vi "采配水流程与超标留样交互.vi"(11 "参数":T1) -> ()   [LabVIEW 2016, in "PLC.lvlib"]
uses:
  PLC.lvlib
panel:
  out "输出数组":cluster{"参数名":string, "浓度":dbl}[](array[cluster])
  out "数值":i32
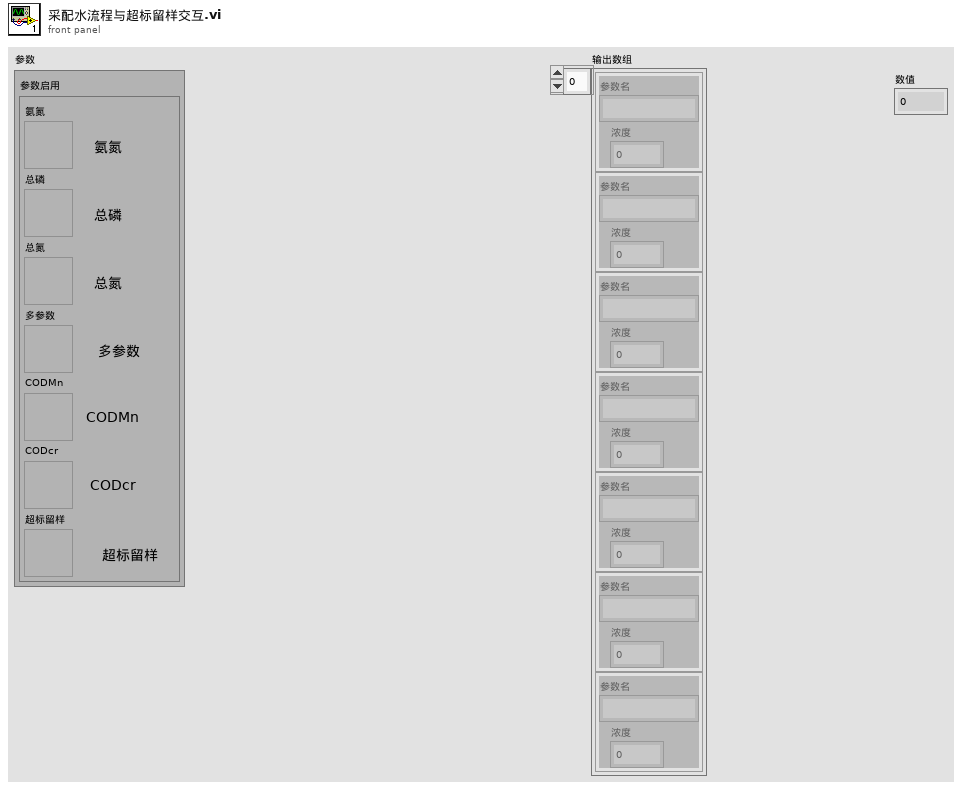
[diagram p1: front panel]
types:
  T1 = cluster{"参数启用":cluster{"氨氮":bool, "总磷":bool, "总氮":bool, "多参数":bool, "CODMn":bool, "CODcr":bool, "超标留样":bool}}
  T2 = cluster{"因子编码":u32, "单位":u16, "标样参考值":sgl, "水样数据时间":timestamp, "水样实测值":sgl, "水样数据标识":string, "标样数据时间":timestamp, "标样实测值":sgl, "标样数据标识":string, "空白数据时间":timestamp, "空白实测值":sgl, "空白数据标识":string, "零点核查数据时间":timestamp, "零点核查实测值":sgl, "零点核查数据标识":string, "跨度核查数据时间":timestamp, "跨度核查实测值":sgl, "跨度核查数据标识":string, "加标回收数据时间":timestamp, "加标回收实测值":sgl, "加标回收数据标识":string, "平行样数据时间":timestamp, "平行样实测值":sgl, "平行样数据标识":string, "F0":sgl, "F1":sgl, "F2":sgl, "F3":sgl, "F4":sgl, "F5":sgl, "F6":sgl, "F7":sgl, "温度":sgl, "湿度":sgl, "X值":sgl, "fidrange":u16}
  T3 = cluster{"温度测量值":sgl, "测量值":sgl, "温度偏移修正值":sgl, "信号值":sgl, "数据标识":string}
  T4 = cluster{"温度测量值":sgl, "DO%":sgl, "DOmg/L":sgl, "温度偏移修正值":sgl, "数据标识mg/L":string, "数据标识%":string}
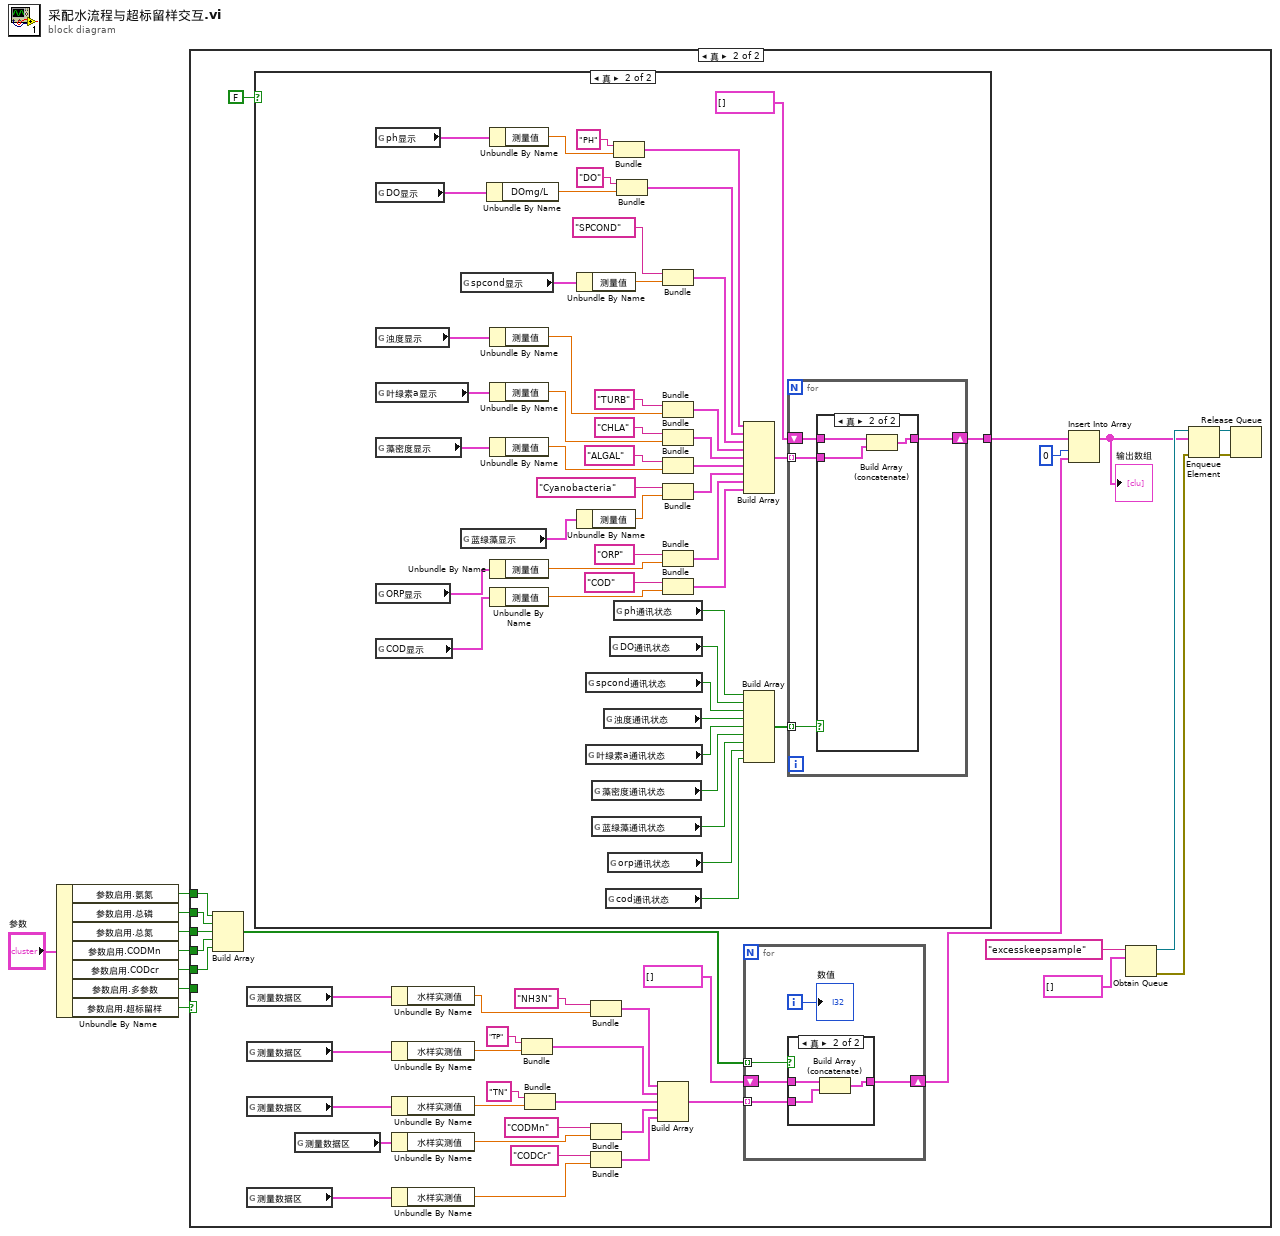
[diagram p0: block diagram]
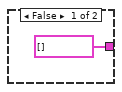
[diagram p4: hidden frame]
diagram:
  n1 = Unbundle By Name("参数") -> ("参数启用.氨氮"=w2:bool, "参数启用.总磷"=w3:bool, "参数启用.总氮"=w4:bool, "参数启用.CODMn"=w5:bool, "参数启用.CODcr"=w6:bool, "参数启用.多参数"=w7:bool, "参数启用.超标留样"=w1:bool)
  n2 = case shown="真" w1 {
    tunnel: w7 -> [_ _]
    tunnel: w6 -> [_ w33]
    tunnel: w5 -> [_ w32]
    tunnel: w4 -> [_ w31]
    tunnel: w3 -> [_ w30]
    tunnel: w2 -> [_ w29]
    frame False {
    }
    frame True {
      n3 = Build Array(w29, w30, w31, w32, w33) -> (w28:bool[])
      n4 = global read "VAR总磷总氮全局变量.vi" "测量数据区"() -> (w40:T2)
      n5 = global read "VAR总磷总氮全局变量.vi" "测量数据区"() -> (w35:T2)
      n6 = global read "VAR总磷总氮全局变量.vi" "测量数据区"() -> (w34:T2)
      n7 = global read "VAR总磷总氮全局变量.vi" "测量数据区"() -> (w10:T2)
      n8 = case shown="真" FALSE {
        tunnel: [cluster{"参数名":string, "浓度":dbl}[] [] w58] -> w20
        frame False {
        }
        frame True {
          n9 = global read "多参数全局变量.vi" "ph显示"() -> (w90:T3)
          n10 = global read "多参数全局变量.vi" "DO显示"() -> (w106:T4)
          n11 = global read "多参数全局变量.vi" "浊度显示"() -> (w105:T3)
          n12 = global read "多参数全局变量.vi" "叶绿素a显示"() -> (w102:T3)
          n13 = global read "多参数全局变量.vi" "藻密度显示"() -> (w103:T3)
          n14 = global read "多参数全局变量.vi" "ORP显示"() -> (w101:T3)
          n15 = global read "多参数全局变量.vi" "COD显示"() -> (w100:T3)
          n16 = global read "多参数全局变量.vi" "spcond显示"() -> (w82:T3)
          n17 = global read "多参数全局变量.vi" "蓝绿藻显示"() -> (w104:T3)
          n18 = Unbundle By Name(w106) -> ("DOmg/L"=w85:sgl)
          n19 = Unbundle By Name(w90) -> ("测量值"=w89:sgl)
          n20 = Unbundle By Name(w105) -> ("测量值"=w77:sgl)
          n21 = Unbundle By Name(w102) -> ("测量值"=w74:sgl)
          n22 = Unbundle By Name(w103) -> ("测量值"=w72:sgl)
          n23 = Unbundle By Name(w101) -> ("测量值"=w65:sgl)
          n24 = Unbundle By Name(w100) -> ("测量值"=w64:sgl)
          n25 = Unbundle By Name(w82) -> ("测量值"=w81:sgl)
          n26 = Unbundle By Name(w104) -> ("测量值"=w66:sgl)
          n27 = global read "多参数全局变量.vi" "spcond通讯状态"() -> (w97:bool)
          n28 = global read "多参数全局变量.vi" "叶绿素a通讯状态"() -> (w95:bool)
          n29 = global read "多参数全局变量.vi" "藻密度通讯状态"() -> (w94:bool)
          n30 = global read "多参数全局变量.vi" "蓝绿藻通讯状态"() -> (w93:bool)
          n31 = global read "多参数全局变量.vi" "浊度通讯状态"() -> (w96:bool)
          n32 = global read "多参数全局变量.vi" "cod通讯状态"() -> (w91:bool)
          n33 = global read "多参数全局变量.vi" "orp通讯状态"() -> (w92:bool)
          n34 = global read "多参数全局变量.vi" "DO通讯状态"() -> (w98:bool)
          n35 = Bundle("PH", "测量值"=w89) -> (w86:cluster{string, "测量值":sgl})  [unwired: 1 in]
          n36 = global read "多参数全局变量.vi" "ph通讯状态"() -> (w99:bool)
          n37 = Bundle("DO", "DOmg/L"=w85) -> (w83:cluster{string, "DOmg/L":sgl})  [unwired: 1 in]
          n38 = Bundle("SPCOND", "测量值"=w81) -> (w79:cluster{string, "测量值":sgl})  [unwired: 1 in]
          n39 = Bundle("TURB", "测量值"=w77) -> (w76:cluster{string, "测量值":sgl})  [unwired: 1 in]
          n40 = Bundle("CHLA", "测量值"=w74) -> (w71:cluster{string, "测量值":sgl})  [unwired: 1 in]
          n41 = Bundle("ALGAL", "测量值"=w72) -> (w70:cluster{string, "测量值":sgl})  [unwired: 1 in]
          n42 = Bundle("Cyanobacteria", "测量值"=w66) -> (w63:cluster{string, "测量值":sgl})  [unwired: 1 in]
          n43 = Bundle("ORP", "测量值"=w65) -> (w62:cluster{string, "测量值":sgl})  [unwired: 1 in]
          n44 = Bundle("COD", "测量值"=w64) -> (w61:cluster{string, "测量值":sgl})  [unwired: 1 in]
          n45 = Build Array(w86, w83, w79, w76, w71, w70, w63, w62, w61) -> (w60:cluster{string, "测量值":sgl}[])
          n46 = Build Array(w99, w98, w97, w96, w95, w94, w93, w92, w91) -> (w59:bool[])
          n47 = for {
            shift-right: [w109] -> w58
            shift-left: cluster{"参数名":string, "浓度":dbl}[] [] -> [w110]
            tunnel: w60 -> [w108] mode=indexing
            tunnel: w59 -> [w107] mode=indexing
            n48 = case shown="真" w107 {
              tunnel: w110 -> [w111 w114]
              tunnel: [w111 w113] -> w109
              tunnel: w108 -> [_ w112]
              frame False {
              }
              frame True {
                n49 = Build Array (concatenate)(w114, w112) -> (w113:cluster{"参数名":string, "浓度":dbl}[])
              }
            }
          }
        }
      }
      n50 = global read "VARCODMn全局变量.vi" "测量数据区"() -> (w46:T2)
      n51 = Unbundle By Name(w40) -> ("水样实测值"=w42:sgl)
      n52 = Unbundle By Name(w35) -> ("水样实测值"=w38:sgl)
      n53 = Unbundle By Name(w34) -> ("水样实测值"=w37:sgl)
      n54 = Unbundle By Name(w46) -> ("水样实测值"=w45:sgl)
      n55 = Unbundle By Name(w10) -> ("水样实测值"=w43:sgl)
      n56 = Bundle("TP", "水样实测值"=w38) -> (w25:cluster{string, "水样实测值":sgl})  [unwired: 1 in]
      n57 = Bundle("TN", "水样实测值"=w37) -> (w24:cluster{string, "水样实测值":sgl})  [unwired: 1 in]
      n58 = Bundle("NH3N", "水样实测值"=w42) -> (w26:cluster{string, "水样实测值":sgl})  [unwired: 1 in]
      n59 = Bundle("CODMn", "水样实测值"=w45) -> (w23:cluster{string, "水样实测值":sgl})  [unwired: 1 in]
      n60 = Bundle("CODCr", "水样实测值"=w43) -> (w22:cluster{string, "水样实测值":sgl})  [unwired: 1 in]
      n61 = Build Array(w26, w25, w24, w23, w22) -> (w21:cluster{string, "水样实测值":sgl}[])
      n62 = for {
        tunnel: w28 -> [w49] mode=indexing
        shift-right: [w50] -> w18
        shift-left: cluster{"参数名":string, "浓度":dbl}[] [] -> [w52]
        tunnel: w21 -> [w51] mode=indexing
        i -> [w48]
        n63 = case shown="真" w49 {
          tunnel: w52 -> [w53 w56]
          tunnel: w51 -> [_ w55]
          tunnel: [w53 w54] -> w50
          frame False {
          }
          frame True {
            n64 = Build Array (concatenate)(w56, w55) -> (w54:cluster{"参数名":string, "浓度":dbl}[])
          }
        }
        "数值" <- w48
      }
      n65 = Insert Into Array(array=w20, index=0 ("索引"), new element=w18) -> (w11:cluster{"参数名":string, "浓度":dbl}[])
      "输出数组" <- w11
      n66 = Obtain Queue(name (unnamed)="excesskeepsample" ("名称（未命名）"), element data type=cluster{"参数名":string, "浓度":dbl}[] []) -> (queue out=w15:refnum<queue>, error out=w14:errorcluster)  [unwired: 3 in, 1 out]
      n67 = Enqueue Element(queue=w15, element=w11, error in (no error)=w14) -> (queue out=w13:refnum<queue>, error out=w12:errorcluster)  [unwired: 1 in, 1 out]
      n68 = Release Queue(queue=w13, error in (no error)=w12) -> ()  [unwired: 1 in, 3 out]
    }
  }
